vi "tiff stack write module.vi"(2 "Compression Type (None)":i32(ring) items=["None", "JPEG", "Run Length Encoded", "Zip"], 3 "Array of Images (U8, U16, I16)":T1[](array[typedef]), 4 "Show Progress? (T)":bool=TRUE, 5 "action":enum16{"open", "save", "close"}(ring)=enum."close", 6 "Add metadata? (T)":bool=TRUE, 7 "i":dbl, 8 "error in":errorcluster, 10 "Convert to U16?":bool, 11 "ImageDescriptions":string[](array[string])) -> (0 "error out":errorcluster)   [LabVIEW 2018]
uses:
  <vilib>/vision/Image Controls.llb/IMAQ Image.ctl
  <vilib>/vision/NI_Vision_Development_Module.lvlib
  Dans Tiff Stack Code/File IO/Image/Tiff/Tiff reader.lvlib
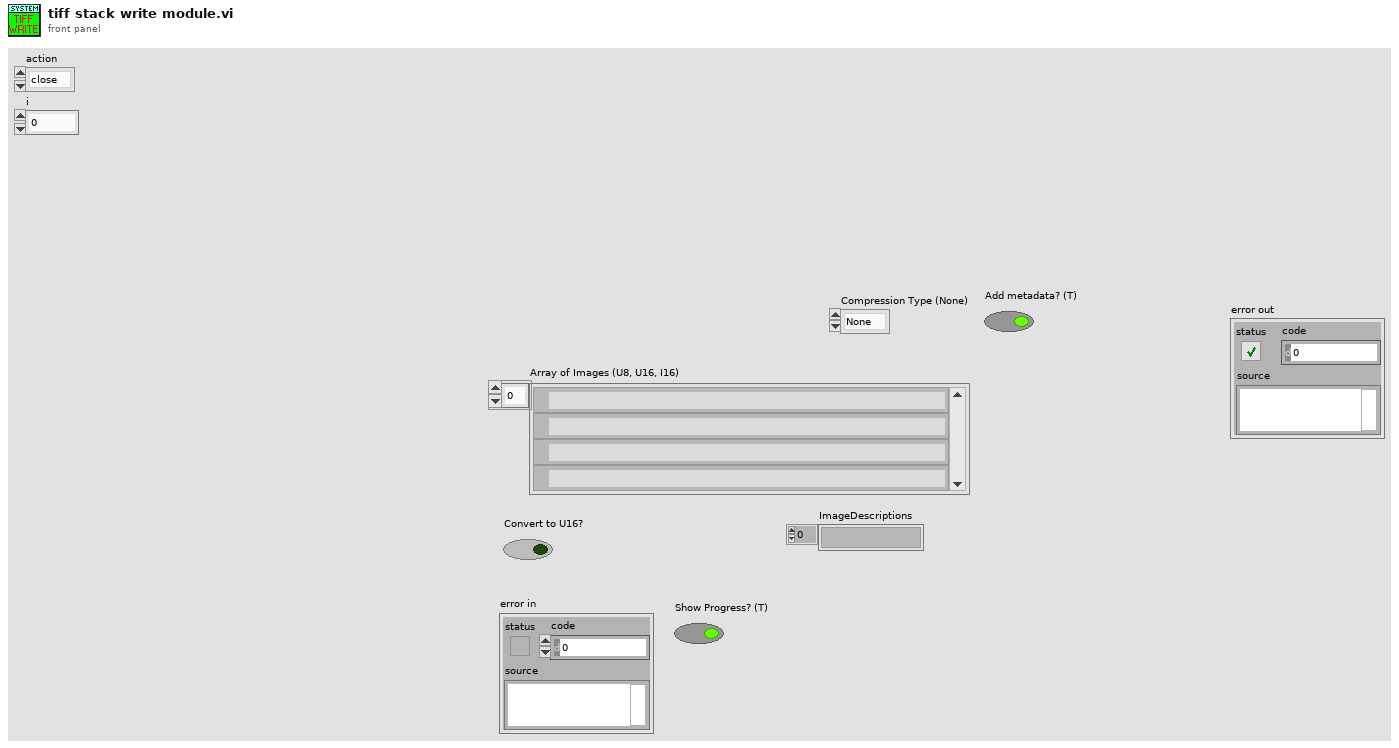
[diagram p1: front panel]
types:
  T1 = typedef "IMAQ Image.ctl" = refnum<image>
  T2 = cluster{"Rows Per Strip":i32, "Photometric":i32, "Compression Type":i32}
  T3 = enum16{"open", "replace", "create", "open or create", "replace or create", "replace or create with confirmation"}
  T4 = typedef "Image Type" = u32
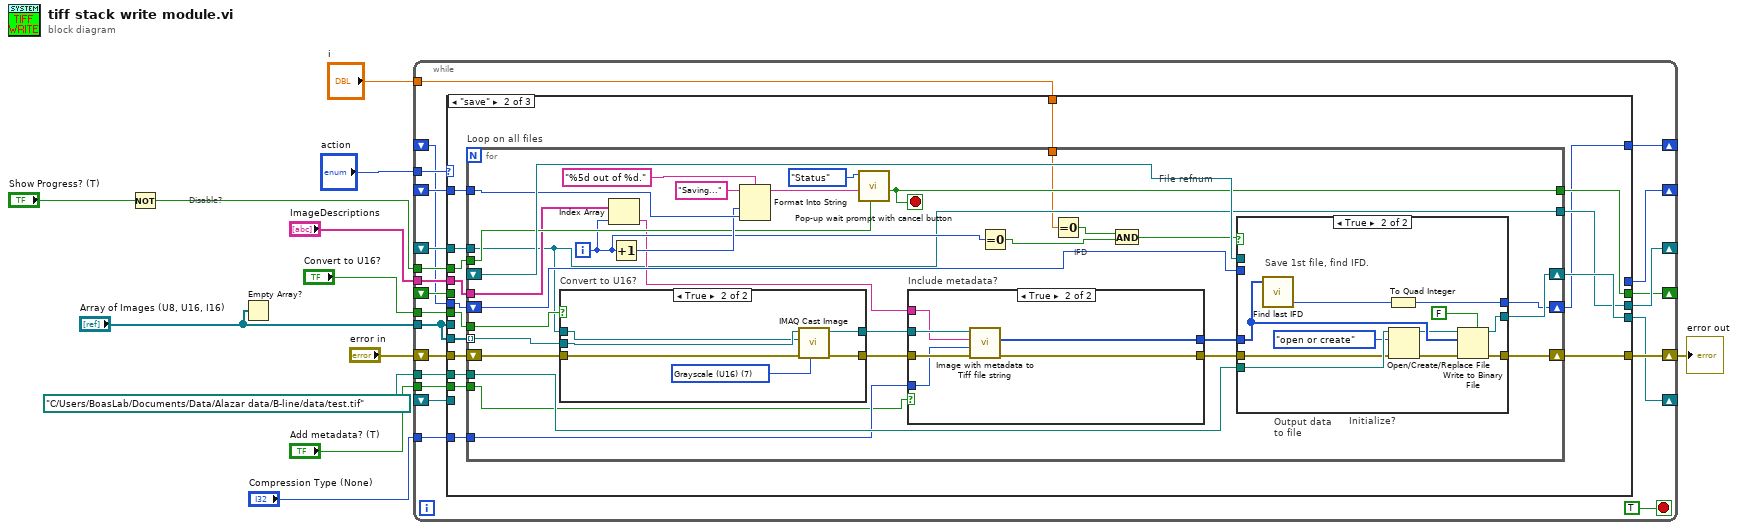
[diagram p0: block diagram]
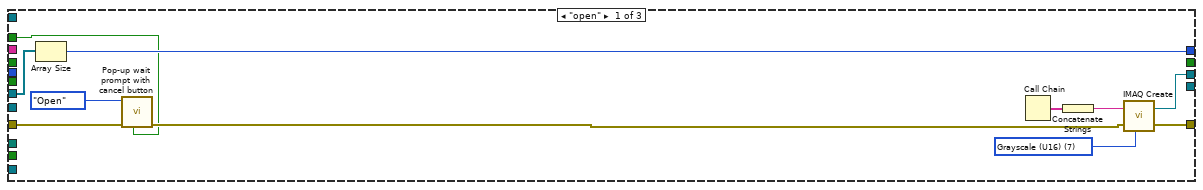
[diagram p2: hidden frame]
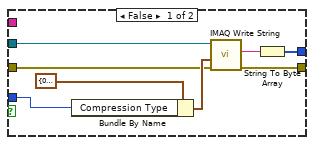
[diagram p3: hidden frame]
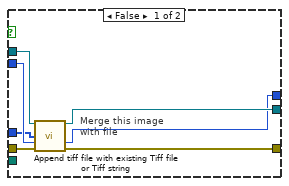
[diagram p5: hidden frame]
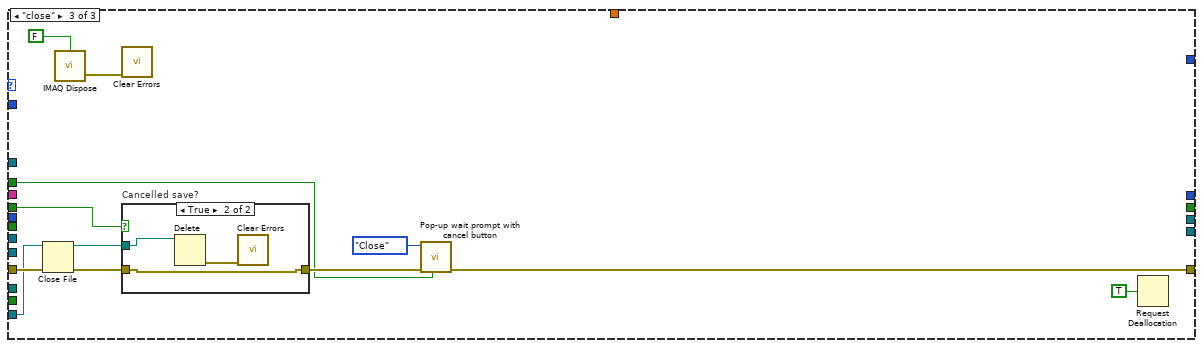
[diagram p6: hidden frame]
diagram:
  # "Disable?"
  n1 = Not(x="Show Progress? (T)") -> (.not. x?=w5:bool)
  n2 = Empty Array?(array="Array of Images (U8, U16, I16)") -> ()  [unwired: 1 out]
  n3 = while {
    tunnel: "Array of Images (U8, U16, I16)" -> [w28]
    tunnel: "Add metadata? (T)" -> [w25]
    tunnel: path "C:/Users/BoasLab/Documents/Data/Alazar data/B-line/data/test.tif" ("Path") -> [w26]
    tunnel: "ImageDescriptions" -> [w27]
    tunnel: "Convert to U16?" -> [w24]
    tunnel: w5 -> [w23]
    tunnel: "Compression Type (None)" -> [w21]
    tunnel: "action" -> [w34]
    shift-right: [w32] -> w2
    shift-left: "error in" -> [w31]
    shift-right: [w30] -> _
    shift-left: _ -> [w29]
    shift-right: [w33] -> _
    shift-left: _ -> [w22]
    shift-right: [w20] -> _
    shift-left: _ -> [w19]
    shift-right: [w18] -> _
    shift-left: _ -> [w17]
    shift-right: [w15] -> _
    shift-left: _ -> [w14]
    tunnel: "i" -> [w13]
    stop <- TRUE stop-if-true
    n4 = case shown="\"save\"" w34 {
      tunnel: [w40 w50 w134] -> w32
      tunnel: w28 -> [w39 _ _]
      tunnel: [w38 _ _] -> w33
      tunnel: w31 -> [w37 w57 w138]
      tunnel: [w36 w49 _] -> w30
      tunnel: w29 -> [_ w62 _]
      tunnel: w28 -> [_ w61 _]
      tunnel: w27 -> [_ w60 _]
      tunnel: w26 -> [_ w59 _]
      tunnel: w25 -> [_ w58 _]
      tunnel: w24 -> [_ w56 _]
      tunnel: w23 -> [w35 w55 w135]
      tunnel: w22 -> [_ w54 _]
      tunnel: w21 -> [_ w53 _]
      tunnel: [_ w52 _] -> w20
      tunnel: w19 -> [_ _ w137]
      tunnel: [_ w51 _] -> w18
      tunnel: w17 -> [_ _ w136]
      tunnel: [_ w48 _] -> w15
      tunnel: w14 -> [_ w47 _]
      tunnel: w13 -> [_ w46 _]
      frame "open" {
        w44 = T4 7 items=["Grayscale (U8)", "Grayscale (I16)", "Grayscale (SGL)", "Complex (CSG)", "RGB (U32)", "HSL (U32)", "RGB (U64)", "Grayscale (U16)"] ("Image Type")
        n5 = Array Size(array=w39) -> (size(s)=w38:i32)
        n6 = call "Pop-up wait prompt with cancel button.vi"("Disable? (F)"=w35, "error in"=w37, "Control"=enum16{"Open", "Close", "Status", "No Change"}."Open") -> ("error out"=w43:errorcluster)  [unwired: 2 in, 6 out]
        n7 = Call Chain() -> (call chain=w42:string[])
        n8 = Concatenate Strings(w42) -> (w41:string)
        n9 = call "IMAQ Create"("Image Name"=w41, "Image Type"=w44, "error in (no error)"=w43) -> ("New Image"=w36:T1, "error out"=w40:errorcluster)  [unwired: 1 in, 1 out]
      }
      frame "save" {
        n10 = for "Loop on all files" {
          tunnel: w61 -> [w82] mode=indexing
          tunnel: w59 -> [w93]
          shift-right: [w92] -> w50
          shift-left: w57 -> [w83]
          shift-right: [w91] -> w52
          shift-left: _ -> [w90]
          shift-right: [w88] -> w48
          shift-left: w47 -> [w89]
          tunnel: w54 -> [w85]
          tunnel: w62 -> [w67]
          tunnel: w56 -> [w81]
          tunnel: [w78] -> w51
          tunnel: w55 -> [w73]
          tunnel: w53 -> [w72]
          tunnel: w58 -> [w71]
          tunnel: w60 -> [w69]
          tunnel: [w67] -> w49
          tunnel: w46 -> [w64]
          i -> [w70]
          stop <- w78 stop-if-true
          # "File refnum"
          # "IFD"
          # "Output data\nto file"
          n11 = case "Convert to U16?" shown="True" w81 {
            tunnel: w83 -> [w108 w115]
            tunnel: [w108 w114] -> w76
            tunnel: w82 -> [w109 w113]
            tunnel: w67 -> [_ w112]
            tunnel: [w109 w110] -> w77
            frame False {
            }
            frame True {
              w111 = T4 7 items=["Grayscale (U8)", "Grayscale (I16)", "Grayscale (SGL)", "Complex (CSG)", "RGB (U32)", "HSL (U32)", "RGB (U64)", "Grayscale (U16)"] ("Image Type")
              n12 = call "IMAQ Cast Image"("Image Type"=w111, "error in (no error)"=w115, "Image Dst"=w112, "Image Src"=w113) -> ("error out"=w114:errorcluster, "Image Dst Out"=w110:T1)  [unwired: 2 in, 4 out]
            }
          }
          n13 = Index Array(array=w69, index=w70) -> (element=w68:string)
          n14 = Increment(x=w70) -> (x+1=w84:i32)
          n15 = Format Into String(format string="%5d out of %d.", initial string="Saving..." ("Prompt Text"), w84, w85) -> (resulting string=w79:string)  [unwired: 1 in, 1 out]
          n16 = call "Pop-up wait prompt with cancel button.vi"("Disable? (F)"=w73, "Prompt Text"=w79, "Control"=enum16{"Open", "Close", "Status", "No Change"}."Status") -> ("Cancel"=w78:bool)  [unwired: 2 in, 6 out]
          n17 = case "Include metadata?" shown="True" w71 {
            tunnel: w77 -> [w96 w107]
            tunnel: w76 -> [w97 w106]
            tunnel: [w98 w105] -> w75
            tunnel: [w94 w104] -> w74
            tunnel: w72 -> [w95 w103]
            tunnel: w68 -> [_ w102]
            frame False {
              n18 = Bundle By Name(cluster=T2 {"Rows Per Strip"=0, "Photometric"=1, "Compression Type"=0} ("TIFF Options"), "Compression Type"=w95) -> (w100:T2)
              n19 = call-poly "IMAQ Write String"("error in (no error)"=w97, "TIFF Options"=w100, "Image"=w96) -> ("error out"=w98:errorcluster, "FileString"=w99:string)  [unwired: 2 in, 5 out]
              n20 = String To Byte Array(string=w99) -> (unsigned byte array=w94:u8[])
            }
            frame True {
              n21 = call "Image with metadata to Tiff file string.vi"("error in"=w106, "Compression Type (None)"=w103, "ImageDescription string\n(must be at least 5 char long)"=w102, "img"=w107) -> ("error out"=w105:errorcluster, "Tiff file out (unsigned byte array)"=w104:u8[])  [unwired: 2 out]
            }
          }
          n22 = Equal To 0?(x=w70) -> (x = 0?=w65:bool)
          n23 = Equal To 0?(x=w64) -> (x = 0?=w66:bool)
          n24 = And(x=w66, y=w65) -> (x .and. y?=w63:bool)
          n25 = case "Initialize?" shown="True" w63 {
            tunnel: w75 -> [w121 w125]
            tunnel: w93 -> [_ w127]
            tunnel: [w122 w133] -> w92
            tunnel: [w119 w132] -> w91
            tunnel: w90 -> [w120 _]
            tunnel: w89 -> [w118 _]
            tunnel: [w117 w129] -> w88
            tunnel: w74 -> [w116 w128]
            frame False {
              # "Merge this image\nwith file"
              n26 = call "Append tiff file with existing Tiff file or Tiff string.vi"("Existing Tiff File (A) refnum"=w120, "Tiff file (B)\n (unsigned byte array)"=w116, "Location in existing file of\nit's last page's \n\"next IFD pointer\""=w118, "error in"=w121) -> ("File refnum out"=w119:refnum<file>, "Location in new file of\nit's last page's \n\"next IFD pointer\""=w117:i64, "error out"=w122:errorcluster)  [unwired: 3 in, 6 out]
            }
            frame True {
              # "Save 1st file, find IFD."
              n27 = call "Find last IFD.vi"("TIFF Data in"=w128) -> ("Location in byte stream of last IFD pointer.  This\nis the word to change if you are adding another page\nto the file."=w130:i32)  [unwired: 4 out]
              n28 = To Quad Integer(1:w130) -> (0:w129:i64)
              n29 = Open/Create/Replace File(file path (use dialog)=w127, error in=w125, operation (0:open)=T3."open or create") -> (refnum out=w123:refnum<file>, error out=w124:errorcluster)  [unwired: 3 in, 1 out]
              n30 = Write to Binary File(file (use dialog)=w123, data=w128, error in=w124, 5:FALSE ("prepend array or string size? (T)")) -> (refnum out=w132:refnum<file>, error out=w133:errorcluster)  [unwired: 1 in, 2 out]
            }
          }
        }
      }
      frame "close" {
        n31 = Close File(refnum=w137, error in=w138) -> (path=w142:path, error out=w143:errorcluster)
        n32 = call "IMAQ Dispose"("All Images? (No)"=FALSE) -> ("error out"=w144:errorcluster)  [unwired: 2 in, 3 out]
        n33 = call <vilib>:"Clear Errors.vi"("error in (no error)"=w144) -> ()  [unwired: 1 in, 6 out]
        n34 = case "Cancelled save?" shown="True" w136 {
          tunnel: w143 -> [w146 w147]
          tunnel: w142 -> [_ w149]
          tunnel: [w146 w147] -> w141
          frame False {
          }
          frame True {
            n35 = Delete(path (use dialog)=w149) -> (error out=w148:errorcluster)  [unwired: 1 in, 5 out]
            n36 = call <vilib>:"Clear Errors.vi"("error in (no error)"=w148) -> ()  [unwired: 1 in, 6 out]
          }
        }
        n37 = call "Pop-up wait prompt with cancel button.vi"("Disable? (F)"=w135, "error in"=w141, "Control"=enum16{"Open", "Close", "Status", "No Change"}."Close") -> ("error out"=w134:errorcluster)  [unwired: 2 in, 6 out]
        n38 = Request Deallocation(TRUE ("flag")) -> ()
      }
    }
  }
  "error out" <- w2
